vi "Testconandread.vi"() -> ()   [LabVIEW 2018]
panel:
  out "read buffer":string
  in  "baud rate (9600)":u32=9600
  in  "VISA resource name":refnum<visa-resource-name>
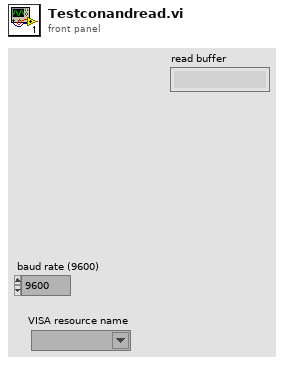
[diagram p1: front panel]
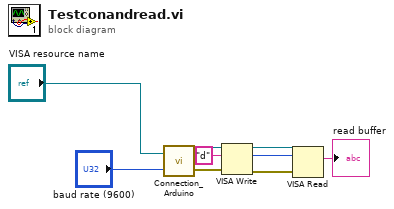
[diagram p0: block diagram]
diagram:
  n1 = call "Connection_Arduino.vi"("baud rate (9600)"="baud rate (9600)", "VISA resource name"="VISA resource name") -> ("error out"=w6:errorcluster, "VISA resource name out"=w7:refnum<visa-resource-name>)
  n2 = VISA Write(VISA resource name=w7, write buffer="d", error in (no error)=w6) -> (VISA resource name out=w4:refnum<visa-resource-name>, return count=w3:u32, error out=w2:errorcluster)
  n3 = VISA Read(VISA resource name=w4, byte count=w3, error in (no error)=w2) -> (read buffer=→"read buffer":string)  [unwired: 3 out]
